vi "ExcelSave.vi"(8 "error in":errorcluster, 10 "Selection Size":T1={"Row"=110, "Column"=6}, 11 "Table in":refnum<vi>) -> (0 "error out":errorcluster)   [LabVIEW 2017]
uses:
  <vilib>/Utility/miscctls.llb/LVRowAndColumnTypeDef.ctl
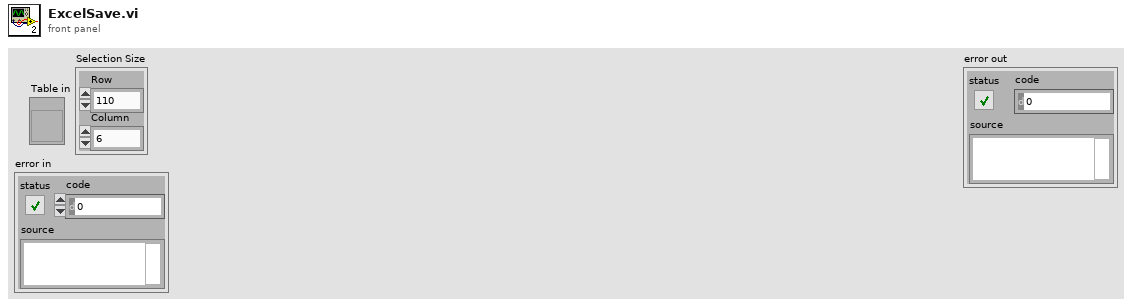
[diagram p1: front panel]
types:
  T1 = typedef "LVRowAndColumnTypeDef.ctl" = cluster{"Row":i32, "Column":i32}
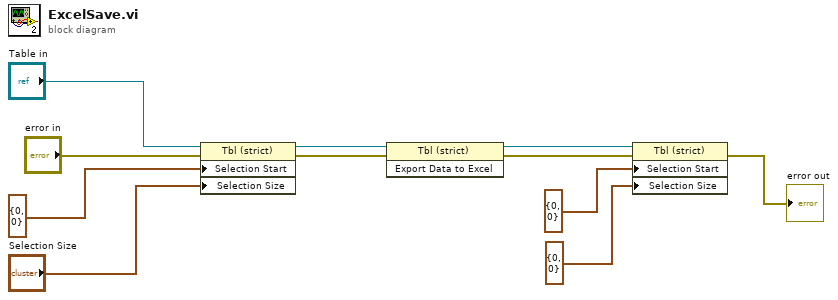
[diagram p0: block diagram]
diagram:
  n1 = property on="Property Node" class="Tbl (strict)"(reference="Table in", error in="error in", "Selection Start"=T1 {"Row"=0, "Column"=0} ("Active Cell:Active Cell"), "Selection Size"="Selection Size") -> (reference out=w11:refnum<vi>, error out=w4:errorcluster)
  n2 = invoke on="Invoke Node" class="Tbl (strict)" method="Export Data to Excel"(reference=w11, error in=w4) -> (reference out=w10:refnum<vi>, error out=w3:errorcluster)  [unwired: 1 in, 1 out]
  n3 = property on="Property Node" class="Tbl (strict)"(reference=w10, error in=w3, "Selection Start"=T1 {"Row"=0, "Column"=0} ("Active Cell:Active Cell"), "Selection Size"=T1 {"Row"=0, "Column"=0}) -> (error out=→"error out":errorcluster)  [unwired: 1 out]
